vi "DSF.Engine.Plugin.Set Debug Flags.vi"(10 "Debug Flags":refnum<class "DSF.Engine.Debug Flags.lvclass">, 11 "Plugin in":refnum<class "DSF.Engine.Plugin.lvclass">) -> (3 "Plugin out":refnum<class "DSF.Engine.Plugin.lvclass">)   [LabVIEW 2017, in "DSF.Engine.lvlib" / "DSF.Engine.Plugin.lvclass"]
uses:
  DSF.Engine.Plugin.lvclass
  Debug/DSF.Engine.Debug Flags.lvclass
  DSF.Engine.Plugin.lvclass/DSF.Engine.Plugin.ctl
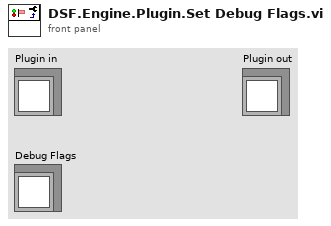
[diagram p1: front panel]
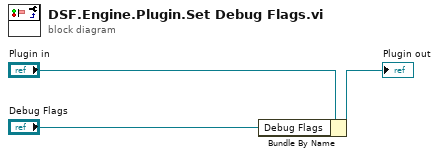
[diagram p0: block diagram]
diagram:
  n1 = Bundle By Name(cluster="Plugin in", "Debug Flags"="Debug Flags") -> (→"Plugin out":refnum<class "DSF.Engine.Plugin.lvclass">)
